vi "Actuate.vi"(0 "Dual Cylinder Actuator in":refnum<class "Dual Cylinder Actuator.lvclass">, 5 "FC1 ILC in":refnum<class "ILC.lvclass">, 7 "FC2 ILC in":refnum<class "ILC.lvclass">, 9 "Actuate Settings":T2 {"FC2 Measured Value" format="%.3f"; "Lateral Demand" format="%.3f"; "FC1 Measured Value" format="%.3f"; "Axial Demand" format="%.3f"}, 11 "error in (no error)":errorcluster) -> (4 "Dual Cylinder Actuator out":refnum<class "Dual Cylinder Actuator.lvclass">, 6 "FC1 ILC out":refnum<class "ILC.lvclass">, 8 "FC2 ILC out":refnum<class "ILC.lvclass">, 10 "Actuate Results":T1 {"FC2 Demand" format="%.3f"; "FC1 Demand" format="%.3f"}, 15 "error out":errorcluster)   [LabVIEW 2015, in "Dual Cylinder Actuator.lvclass"]
uses:
  Dual Cylinder Actuator.lvclass
  <userlib>/Common/ILC/ILC/ILC.lvclass
  Typedefs/Actuate Arguments.ctl
  Typedefs/Actuate Results.ctl
  Dual Cylinder Actuator.lvclass/Dual Cylinder Actuator.ctl
  Actuator Cylinder/Actuator Cylinder/Actuator Cylinder.lvclass
  Typedefs/FAMT Typedefs.lvlib
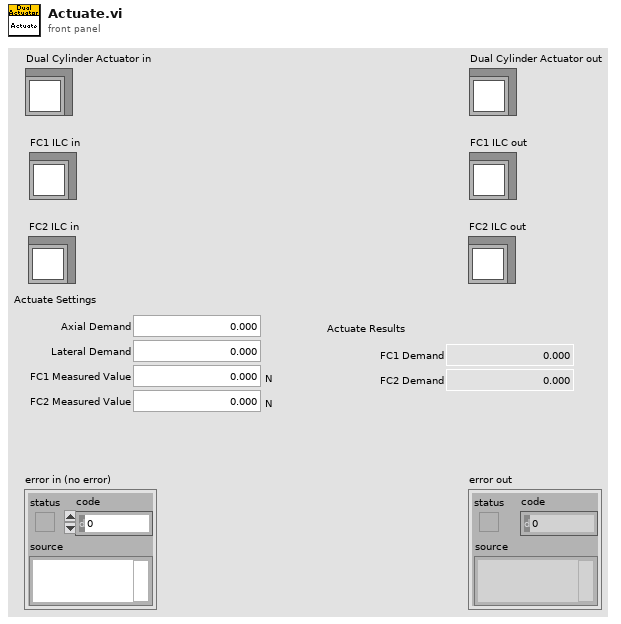
[diagram p1: front panel]
types:
  T1 = typedef "FAMT Typedefs.lvlib/Actuate Results.ctl" = cluster{"FC1 Demand":dbl, "FC2 Demand":dbl}
  T2 = typedef "FAMT Typedefs.lvlib/Actuate Arguments.ctl" = cluster{"Axial Demand":dbl, "Lateral Demand":dbl, "FC1 Measured Value":dbl[unit], "FC2 Measured Value":dbl[unit]}
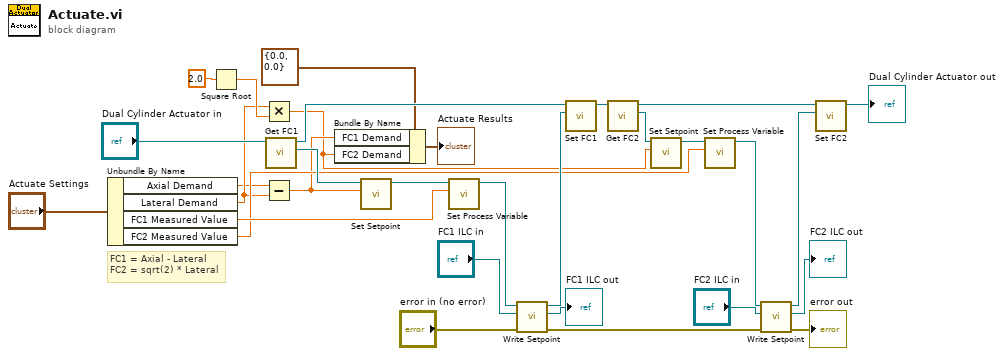
[diagram p0: block diagram]
diagram:
  # "FC1 = Axial - Lateral\nFC2 = sqrt(2) * Lateral"
  n1 = Unbundle By Name("Actuate Settings") -> ("Axial Demand"=w5:dbl, "Lateral Demand"=w6:dbl, "FC1 Measured Value"=w11:dbl[unit], "FC2 Measured Value"=w10:dbl[unit])
  n2 = Square Root(x=2.0) -> (sqrt(x)=w12:dbl)
  n3 = Multiply(x=w6, y=w12) -> (x*y=w1:dbl)
  n4 = Subtract(x=w5, y=w6) -> (x-y=w2:dbl)
  n5 = call "Get FC1.vi"("SingleCylinderActuator in"="Dual Cylinder Actuator in") -> ("FC1"=w30:refnum<class "Actuator Cylinder.lvclass">, "SingleCylinderActuator out"=w24:refnum<class "Dual Cylinder Actuator.lvclass">)  [unwired: 9 in]
  n6 = Bundle By Name(cluster=T1 {"FC1 Demand"=0.0, "FC2 Demand"=0.0} ("Actuate Results"), "FC1 Demand"=w2, "FC2 Demand"=w1) -> (→"Actuate Results":T1)
  n7 = call-dynamic "Set Setpoint.vi"("Setpoint"=w2, "Actuator Cylinder in"=w30) -> ("Actuator Cylinder out"=w29:refnum<class "Actuator Cylinder.lvclass">)  [unwired: 9 in]
  n8 = call-dynamic "Set Process Variable.vi"("Process Variable"=w11, "Actuator Cylinder in"=w29) -> ("Actuator Cylinder out"=w26:refnum<class "Actuator Cylinder.lvclass">)  [unwired: 9 in]
  n9 = call-dynamic "Write Setpoint.vi"("error in (no error)"="error in (no error)", "ILC in"="FC1 ILC in", "Actuator Cylinder in"=w26) -> ("error out"=w21:errorcluster, "ILC out"=→"FC1 ILC out":refnum<class "ILC.lvclass">, "Actuator Cylinder out"=w25:refnum<class "Actuator Cylinder.lvclass">)  [unwired: 6 in]
  n10 = call "Set FC1.vi"("FC1"=w25, "SingleCylinderActuator in"=w24) -> ("SingleCylinderActuator out"=w23:refnum<class "Dual Cylinder Actuator.lvclass">)  [unwired: 9 in]
  n11 = call "Get FC2.vi"("DualCylinderActuator in"=w23) -> ("FC2"=w18:refnum<class "Actuator Cylinder.lvclass">, "DualCylinderActuator out"=w17:refnum<class "Dual Cylinder Actuator.lvclass">)  [unwired: 9 in]
  n12 = call-dynamic "Set Setpoint.vi"("Setpoint"=w1, "Actuator Cylinder in"=w18) -> ("Actuator Cylinder out"=w19:refnum<class "Actuator Cylinder.lvclass">)  [unwired: 9 in]
  n13 = call-dynamic "Set Process Variable.vi"("Process Variable"=w10, "Actuator Cylinder in"=w19) -> ("Actuator Cylinder out"=w20:refnum<class "Actuator Cylinder.lvclass">)  [unwired: 9 in]
  n14 = call-dynamic "Write Setpoint.vi"("error in (no error)"=w21, "ILC in"="FC2 ILC in", "Actuator Cylinder in"=w20) -> ("error out"=→"error out":errorcluster, "ILC out"=→"FC2 ILC out":refnum<class "ILC.lvclass">, "Actuator Cylinder out"=w16:refnum<class "Actuator Cylinder.lvclass">)  [unwired: 6 in]
  n15 = call "Set FC2.vi"("FC2"=w16, "DualCylinderActuator in"=w17) -> ("DualCylinderActuator out"=→"Dual Cylinder Actuator out":refnum<class "Dual Cylinder Actuator.lvclass">)  [unwired: 9 in]
